vi "Implement Authenticate.vi"(8 "error in (no error)":errorcluster, 10 "Challenge Dict":string, 11 "TicketAuthentactor in":refnum<class "TicketAuthentactor.lvclass">) -> (0 "error out":errorcluster, 1 "Authenticate Dict":string, 2 "Authenticate Signature":string, 3 "TicketAuthentactor out":refnum<class "TicketAuthentactor.lvclass">)   [LabVIEW 2020, in "wamplv.lvlib" / "TicketAuthentactor.lvclass"]
uses:
  TicketAuthentactor.lvclass
  TicketAuthentactor.lvclass/TicketAuthentactor.ctl
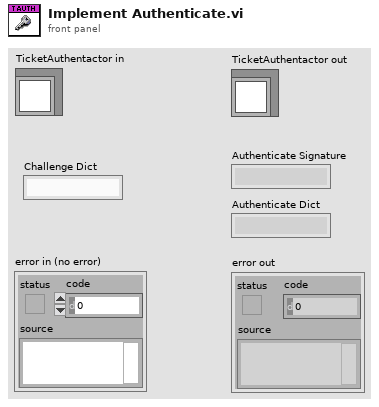
[diagram p1: front panel]
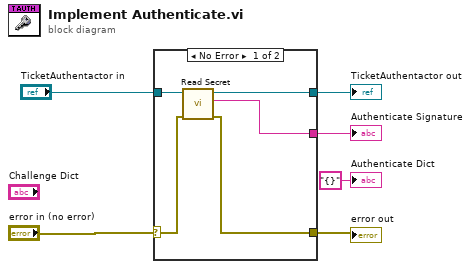
[diagram p0: block diagram]
diagram:
  n1 = case shown="No Error" "error in (no error)" {
    selector: "error in (no error)" -> [w8 w13]
    tunnel: [w7 w13] -> w5
    tunnel: "TicketAuthentactor in" -> [w11 w12]
    tunnel: [w10 w12] -> w3
    tunnel: [w9 _] -> w1
    frame No Error {
      n2 = call-dynamic "Read Secret.vi"("error in (no error)"=w8, "SecretBasedAuthenticatorBase in"=w11) -> ("error out"=w7:errorcluster, "Secret"=w9:string, "SecretBasedAuthenticatorBase out"=w10:refnum<class "TicketAuthentactor.lvclass">)  [unwired: 7 in]
    }
    frame Error {
    }
  }
  "error out" <- w5
  "TicketAuthentactor out" <- w3
  "Authenticate Signature" <- w1
  "Authenticate Dict" <- "{}" ("Authenticate Dict")
